vi "ReadObjectLayout.vi"(7 "properties to ignore":variant, 8 "error in (no error)":errorcluster, 10 "GObj Refnum":refnum<vi>, 11 "Cluster Control Layout in":refnum<class "Cluster Control Layout.lvclass">) -> (0 "error out":errorcluster, 3 "Cluster Control Layout out":refnum<class "Cluster Control Layout.lvclass">)   [LabVIEW 2012, in "NI_SE_Front Panel Layout.lvlib" / "Cluster Control Layout.lvclass"]
doc: "Read layout information from the GObj Refnum."
uses:
  Cluster Control Layout.lvclass
  Control Layout/Control Layout.lvclass
  Object Layout/Object Layout.lvclass
  Cluster Control Layout.lvclass/Cluster Control Layout.ctl
  NI_SE_Front Panel Layout.lvlib
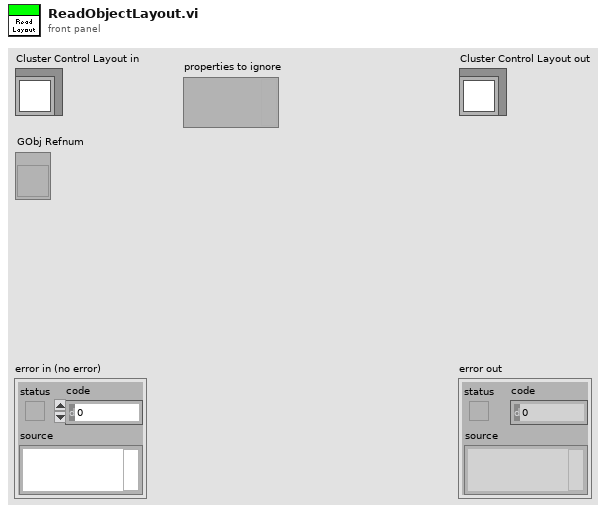
[diagram p1: front panel]
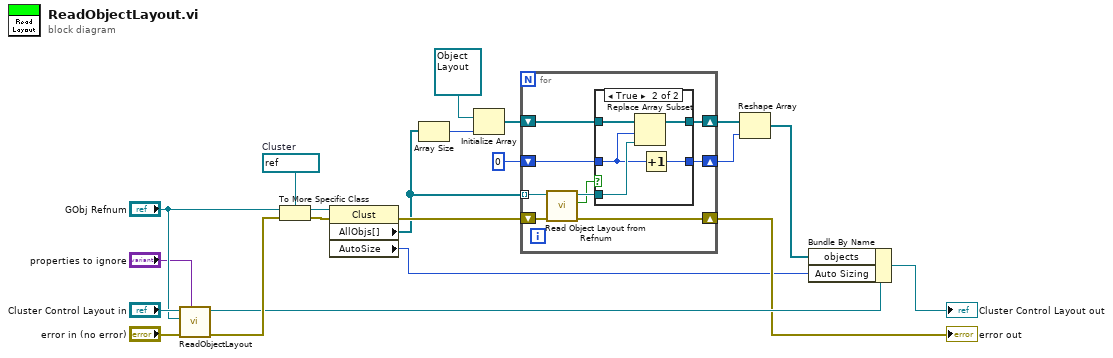
[diagram p0: block diagram]
diagram:
  w13 = refnum<vi> refnum  # Cluster
  n1 = call-parent "ReadObjectLayout.vi"("properties to ignore"="properties to ignore", "error in (no error)"="error in (no error)", "GObj Refnum"="GObj Refnum", "Control Layout in"="Cluster Control Layout in") -> ("error out"=w19:errorcluster, "Control Layout out"=w18:refnum<class "Cluster Control Layout.lvclass">)  [unwired: 6 in]
  n2 = To More Specific Class(target class=w13, reference="GObj Refnum", error in=w19) -> (specific class reference=w12:refnum<vi>, error out=w11:errorcluster)
  n3 = property class="Clust"(reference=w12, error in=w11) -> (error out=w10:errorcluster, "AllObjs[]"=w8:refnum<vi>[], "AutoSize"=w9:u32)  [unwired: 1 out]
  n4 = Array Size(array=w8) -> (size(s)=w6:i32)
  n5 = Initialize Array(refnum<class "Object Layout.lvclass"> refnum ("object layout"), w6) -> (w5:refnum<class "Object Layout.lvclass">[])
  n6 = for {
    tunnel: w8 -> [w30] mode=indexing
    shift-right: [w27] -> w15
    shift-left: w10 -> [w28]
    shift-right: [w24] -> w3
    shift-left: w5 -> [w25]
    shift-right: [w22] -> w1
    shift-left: 0 -> [w23]
    n7 = call "Read Object Layout from Refnum.vi"("error in"=w28, "GObj refnum"=w30) -> ("error out"=w27:errorcluster, "found?"=w26:bool, "object layout"=w29:refnum<class "Object Layout.lvclass">)  [unwired: 7 in]
    n8 = case shown="True" w26 {
      tunnel: w25 -> [w32 w37]
      tunnel: w29 -> [_ w36]
      tunnel: [w32 w35] -> w24
      tunnel: w23 -> [w31 w34]
      tunnel: [w31 w33] -> w22
      frame False {
      }
      frame True {
        n9 = Replace Array Subset(array=w37, new element=w36, index=w34) -> (w35:refnum<class "Object Layout.lvclass">[])
        n10 = Increment(x=w34) -> (x+1=w33:i32)
      }
    }
  }
  "error out" <- w15
  n11 = Reshape Array(w3, w1) -> (w2:refnum<class "Object Layout.lvclass">[])
  n12 = Bundle By Name(cluster=w18, "objects"=w2, "Auto Sizing"=w9) -> (→"Cluster Control Layout out":refnum<class "Cluster Control Layout.lvclass">)
